vi "Read Selected images.vi"(8 "error in (no error)":errorcluster, 11 "HIS in":refnum<class "HIS.lvclass">) -> (0 "error out":errorcluster, 2 "Selected images":i32[](array[numeric]), 3 "HIS out":refnum<class "HIS.lvclass">)   [LabVIEW 2018, in "HIS.lvclass"]
uses:
  HIS.lvclass
  HIS.lvclass/HIS.ctl
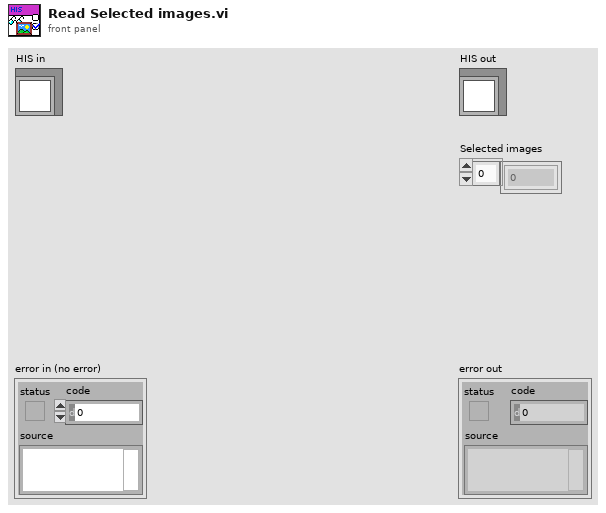
[diagram p1: front panel]
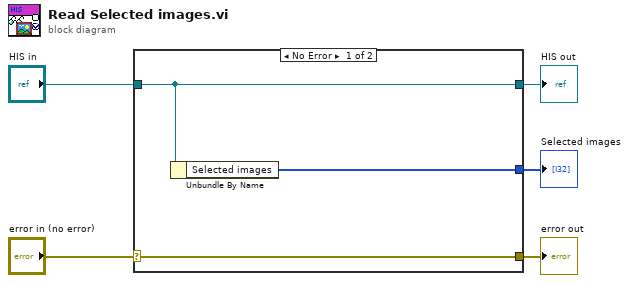
[diagram p0: block diagram]
diagram:
  n1 = case shown="No Error" "error in (no error)" {
    selector: "error in (no error)" -> [w8 w9]
    tunnel: [w8 w9] -> w4
    tunnel: [w7 w10] -> w2
    tunnel: "HIS in" -> [w7 w10]
    tunnel: [w6 _] -> w1
    frame No Error {
      n2 = Unbundle By Name(w7) -> ("Selected images"=w6:i32[])
    }
    frame Error {
    }
  }
  "error out" <- w4
  "HIS out" <- w2
  "Selected images" <- w1
